vi "parse_assembly_state.vi"(0 "Msg in":string, 2 "error in":errorcluster) -> (3 "msg out":string, 4 "Assembly State":T2, 5 "Header":T1, 6 "error out":errorcluster)   [LabVIEW 2012]
uses:
  <userlib>/ROSforLV/ROS/parsing/std_msgs/subs/parse_bool_scalar.vi
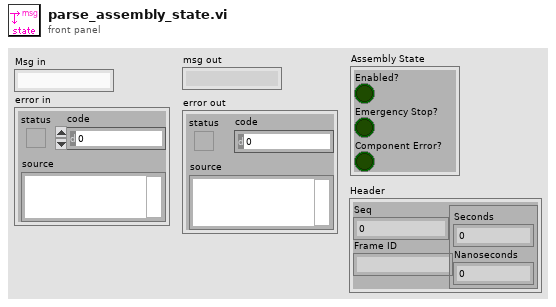
[diagram p1: front panel]
types:
  T1 = cluster{"Seq":u32, "Frame ID":string, "Timestamp":cluster{"Seconds":i32, "Nanoseconds":i32}}
  T2 = cluster{"Enabled?":bool, "Emergency Stop?":bool, "Component Error?":bool}
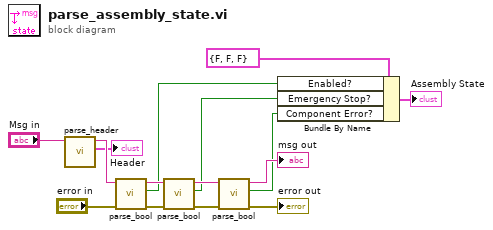
[diagram p0: block diagram]
diagram:
  n1 = call <userlib>:"parse_header.vi"("msg in"="Msg in") -> ("Header"=→"Header":T1, "msg out"=w2:string)  [unwired: 4 in, 1 out]
  n2 = call-poly <userlib>:"parse_bool.vi"("error in"="error in", "msg in"=w2) -> ("error out"=w9:errorcluster, "bool"=w7:bool, "msg out"=w15:string)  [unwired: 3 in]
  n3 = call-poly <userlib>:"parse_bool.vi"("error in"=w9, "msg in"=w15) -> ("error out"=w10:errorcluster, "bool"=w6:bool, "msg out"=w14:string)  [unwired: 3 in]
  n4 = call-poly <userlib>:"parse_bool.vi"("error in"=w10, "msg in"=w14) -> ("error out"=→"error out":errorcluster, "bool"=w5:bool, "msg out"=→"msg out":string)  [unwired: 3 in]
  n5 = Bundle By Name(cluster=T2 {"Enabled?"=FALSE, "Emergency Stop?"=FALSE, "Component Error?"=FALSE} ("input cluster"), "Enabled?"=w7, "Emergency Stop?"=w6, "Component Error?"=w5) -> (→"Assembly State":T2)
